vi "CreateSendMSG.vi"(1 "COM Data":T1, 2 "Controls":u8[](array[numeric])) -> ()   [LabVIEW 2013]
panel:
  out "status":bool
  out "error out":errorcluster
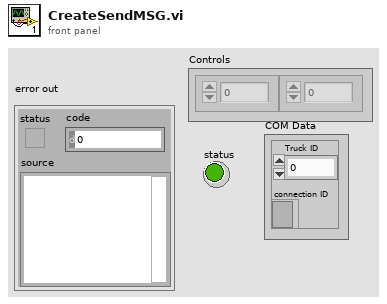
[diagram p1: front panel]
types:
  T1 = cluster{"Truck ID":dbl, "connection ID":refnum<k5>}
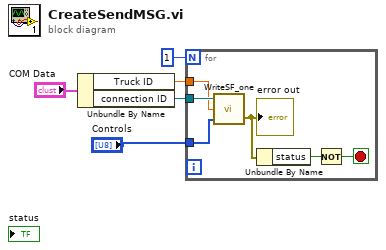
[diagram p0: block diagram]
diagram:
  n1 = Unbundle By Name("COM Data") -> ("Truck ID"=w2:dbl, "connection ID"=w3:refnum<k5>)
  n2 = for {
    N: 1 -> [_]
    tunnel: "Controls" -> [w11]
    tunnel: w3 -> [w10]
    tunnel: w2 -> [w9]
    stop <- w6 stop-if-true
    n3 = call "WriteSF_one.vi"("payload"=w11, "destination ID"=w9, "connection ID in"=w10) -> ("error out"=w8:errorcluster)  [unwired: 1 out]
    "error out" <- w8
    n4 = Unbundle By Name(w8) -> ("status"=w7:bool)
    n5 = Not(x=w7) -> (.not. x?=w6:bool)
  }
